vi "Imposta settings grafico.vi"(9 "Reiniz nome plot":bool, 10 "GRAFICO":T1 {"ASSE Y 5"."Decimali" min=0 max=6; "ASSE Y 4"."Decimali" min=0 max=6; "ASSE Y 3"."Decimali" min=0 max=6; "ASSE Y 2"."Decimali" min=0 max=6; "ASSE Y 1"."Decimali" min=0 max=6; "ASSE X 2"."Decimali" min=0 max=6; "ASSE X 1"."Decimali" min=0 max=6}, 11 "XYGraph in":refnum<vi>) -> ()   [LabVIEW 2019]
uses:
  TypeDef/Definizione_Grafico_REPORT.ctl
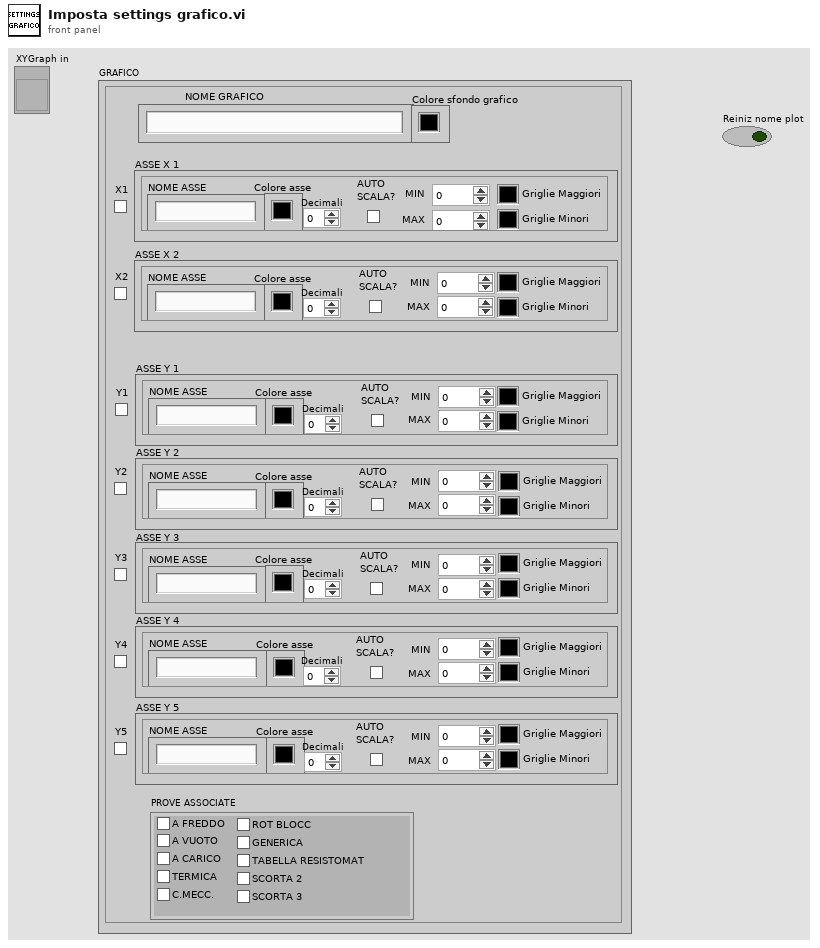
[diagram p1: front panel]
types:
  T1 = typedef "Definizione_Grafico_REPORT.ctl" = cluster{"ASSE X 1":cluster{"NOME ASSE":string, "AUTO\nSCALA?":bool, "MIN":dbl, "MAX":dbl, "Colore asse":u32, "Griglie Maggiori":u32, "Griglie Minori":u32, "Decimali":i8}, "ASSE X 2":cluster{"NOME ASSE":string, "AUTO\nSCALA?":bool, "MIN":dbl, "MAX":dbl, "Colore asse":u32, "Griglie Maggiori":u32, "Griglie Minori":u32, "Decimali":i8}, "ASSE Y 1":cluster{"NOME ASSE":string, "AUTO\nSCALA?":bool, "MIN":dbl, "MAX":dbl, "Colore asse":u32, "Griglie Maggiori":u32, "Griglie Minori":u32, "Decimali":i8}, "ASSE Y 2":cluster{"NOME ASSE":string, "AUTO\nSCALA?":bool, "MIN":dbl, "MAX":dbl, "Colore asse":u32, "Griglie Maggiori":u32, "Griglie Minori":u32, "Decimali":i8}, "ASSE Y 3":cluster{"NOME ASSE":string, "AUTO\nSCALA?":bool, "MIN":dbl, "MAX":dbl, "Colore asse":u32, "Griglie Maggiori":u32, "Griglie Minori":u32, "Decimali":i8}, "ASSE Y 4":cluster{"NOME ASSE":string, "AUTO\nSCALA?":bool, "MIN":dbl, "MAX":dbl, "Colore asse":u32, "Griglie Maggiori":u32, "Griglie Minori":u32, "Decimali":i8}, "X1":bool, "X2":bool, "Y1":bool, "Y2":bool, "Y3":bool, "Y4":bool, "NOME GRAFICO":string, "PROVE ASSOCIATE":cluster{"A FREDDO":bool, "A VUOTO":bool, "A CARICO":bool, "TERMICA":bool, "C.MECC.":bool, "ROT BLOCC":bool, "GENERICA":bool, "TABELLA RESISTOMAT":bool, "SCORTA 2":bool, "SCORTA 3":bool}, "ASSE Y 5":cluster{"NOME ASSE":string, "AUTO\nSCALA?":bool, "MIN":dbl, "MAX":dbl, "Colore asse":u32, "Griglie Maggiori":u32, "Griglie Minori":u32, "Decimali":i8}, "Y5":bool, "Colore sfondo grafico":u32}
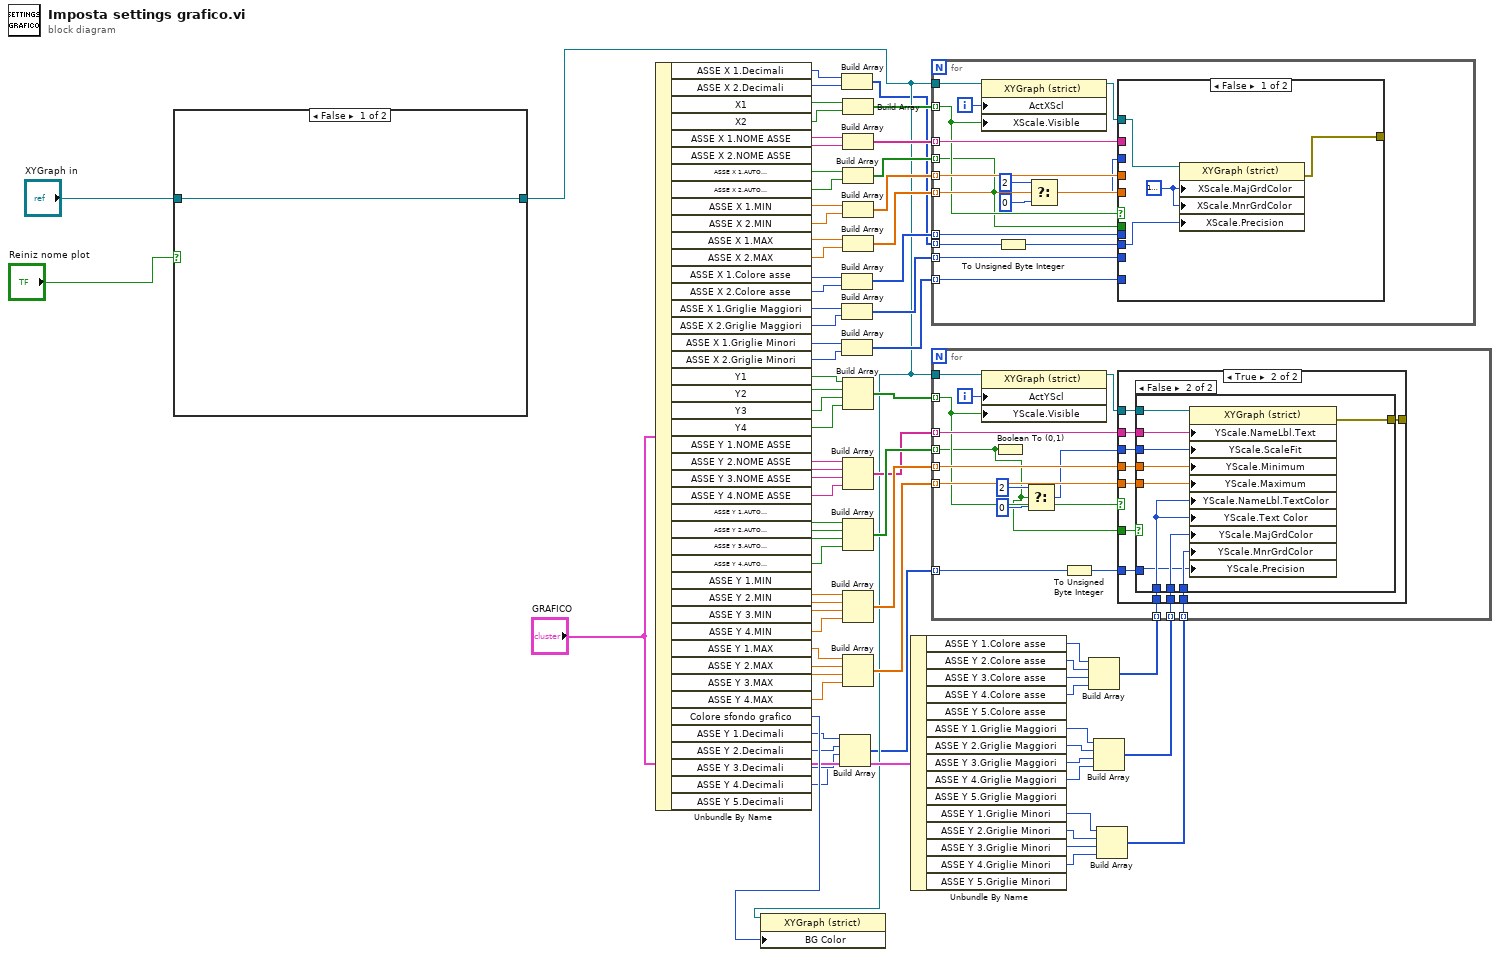
[diagram p0: block diagram]
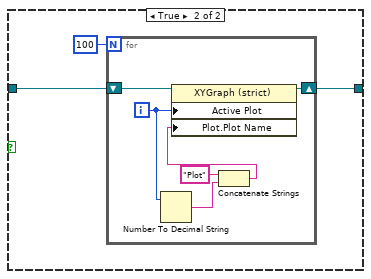
[diagram p2: hidden frame]
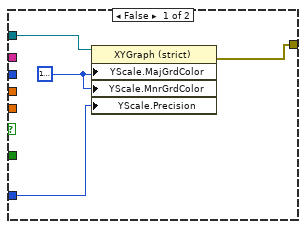
[diagram p3: hidden frame]
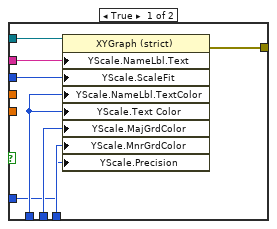
[diagram p4: hidden frame]
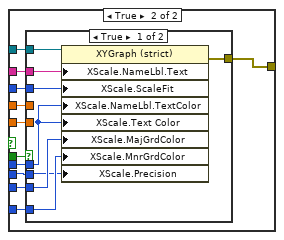
[diagram p5: hidden frame]
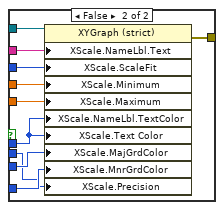
[diagram p6: hidden frame]
diagram:
  n1 = case shown="False" "Reiniz nome plot" {
    tunnel: "XYGraph in" -> [w78 w81]
    tunnel: [w78 w79] -> w7
    frame False {
    }
    frame True {
      n2 = for {
        N: 100 -> [_]
        shift-right: [w82] -> w79
        shift-left: w81 -> [w87]
        i -> [w86]
        n3 = Number To Decimal String(number=w86) -> (decimal integer string=w85:string)  [unwired: 1 in]
        n4 = Concatenate Strings("Plot" ("string"), w85) -> (w83:string)
        n5 = property class="XYGraph (strict)"(reference=w87, "Active Plot"=w86, "Plot.Plot Name"=w83) -> (reference out=w82:refnum<vi>)  [unwired: 1 in, 1 out]
      }
    }
  }
  n6 = Unbundle By Name("GRAFICO") -> ("ASSE X 1.Decimali"=w9:i8, "ASSE X 2.Decimali"=w8:i8, "X1"=w12:bool, "X2"=w13:bool, "ASSE X 1.NOME ASSE"=w15:string, "ASSE X 2.NOME ASSE"=w39:string, "ASSE X 1.AUTO\nSCALA?"=w40:bool, "ASSE X 2.AUTO\nSCALA?"=w41:bool, "ASSE X 1.MIN"=w42:dbl, "ASSE X 2.MIN"=w43:dbl, "ASSE X 1.MAX"=w44:dbl, "ASSE X 2.MAX"=w45:dbl, "ASSE X 1.Colore asse"=w57:u32, "ASSE X 2.Colore asse"=w58:u32, "ASSE X 1.Griglie Maggiori"=w60:u32, "ASSE X 2.Griglie Maggiori"=w61:u32, "ASSE X 1.Griglie Minori"=w63:u32, "ASSE X 2.Griglie Minori"=w64:u32, "Y1"=w59:bool, "Y2"=w20:bool, "Y3"=w21:bool, "Y4"=w22:bool, "ASSE Y 1.NOME ASSE"=w23:string, "ASSE Y 2.NOME ASSE"=w24:string, "ASSE Y 3.NOME ASSE"=w25:string, "ASSE Y 4.NOME ASSE"=w26:string, "ASSE Y 1.AUTO\nSCALA?"=w27:bool, "ASSE Y 2.AUTO\nSCALA?"=w28:bool, "ASSE Y 3.AUTO\nSCALA?"=w29:bool, "ASSE Y 4.AUTO\nSCALA?"=w30:bool, "ASSE Y 1.MIN"=w31:dbl, "ASSE Y 2.MIN"=w32:dbl, "ASSE Y 3.MIN"=w33:dbl, "ASSE Y 4.MIN"=w34:dbl, "ASSE Y 1.MAX"=w35:dbl, "ASSE Y 2.MAX"=w36:dbl, "ASSE Y 3.MAX"=w37:dbl, "ASSE Y 4.MAX"=w38:dbl, "Colore sfondo grafico"=w77:u32, "ASSE Y 1.Decimali"=w1:i8, "ASSE Y 2.Decimali"=w5:i8, "ASSE Y 3.Decimali"=w4:i8, "ASSE Y 4.Decimali"=w3:i8)  [unwired: 1 out]
  n7 = property class="XYGraph (strict)"(reference=w7, "BG Color"=w77) -> ()  [unwired: 1 in, 2 out]
  n8 = Build Array(w1, w5, w4, w3) -> (w2:i8[])
  n9 = Build Array(w9, w8) -> (w6:i8[])
  n10 = Build Array(w57, w58) -> (w51:u32[])
  n11 = Build Array(w60, w61) -> (w62:u32[])
  n12 = Build Array(w63, w64) -> (w65:u32[])
  n13 = Build Array(w12, w13) -> (w14:bool[])
  n14 = Build Array(w15, w39) -> (w16:string[])
  n15 = Build Array(w40, w41) -> (w17:bool[])
  n16 = Build Array(w42, w43) -> (w18:dbl[])
  n17 = Build Array(w44, w45) -> (w19:dbl[])
  n18 = Build Array(w59, w20, w21, w22) -> (w46:bool[])
  n19 = Build Array(w23, w24, w25, w26) -> (w47:string[])
  n20 = Build Array(w27, w28, w29, w30) -> (w48:bool[])
  n21 = Build Array(w31, w32, w33, w34) -> (w49:dbl[])
  n22 = Build Array(w35, w36, w37, w38) -> (w50:dbl[])
  n23 = Unbundle By Name("GRAFICO") -> ("ASSE Y 1.Colore asse"=w53:u32, "ASSE Y 2.Colore asse"=w54:u32, "ASSE Y 3.Colore asse"=w55:u32, "ASSE Y 4.Colore asse"=w56:u32, "ASSE Y 1.Griglie Maggiori"=w66:u32, "ASSE Y 2.Griglie Maggiori"=w67:u32, "ASSE Y 3.Griglie Maggiori"=w68:u32, "ASSE Y 4.Griglie Maggiori"=w69:u32, "ASSE Y 1.Griglie Minori"=w71:u32, "ASSE Y 2.Griglie Minori"=w72:u32, "ASSE Y 3.Griglie Minori"=w73:u32, "ASSE Y 4.Griglie Minori"=w74:u32)  [unwired: 3 out]
  n24 = for {
    tunnel: w14 -> [w97] mode=indexing
    tunnel: w7 -> [w103]
    tunnel: w16 -> [w100] mode=indexing
    tunnel: w17 -> [w92] mode=indexing
    tunnel: w18 -> [w99] mode=indexing
    tunnel: w19 -> [w98] mode=indexing
    tunnel: w51 -> [w96] mode=indexing
    tunnel: w62 -> [w91] mode=indexing
    tunnel: w65 -> [w90] mode=indexing
    tunnel: w6 -> [w89] mode=indexing
    i -> [w102]
    n25 = property class="XYGraph (strict)"(reference=w103, "ActXScl"=w102, "XScale.Visible"=w97) -> (reference out=w101:refnum<vi>)  [unwired: 1 in, 1 out]
    n26 = To Unsigned Byte Integer(number=w89) -> (unsigned 8bit integer=w88:u8)
    n27 = Select(t=i16 2 ("0, 1"), s=w92, f=i16 0 ("0, 1")) -> (s? t:f=w93:i16)
    n28 = case shown="False" w97 {
      tunnel: w101 -> [w107 w118]
      tunnel: w100 -> [_ w117]
      tunnel: w93 -> [_ w116]
      tunnel: w99 -> [_ w115]
      tunnel: w98 -> [_ w114]
      tunnel: w96 -> [_ w113]
      tunnel: w92 -> [_ w112]
      tunnel: w91 -> [_ w111]
      tunnel: w90 -> [_ w110]
      tunnel: w88 -> [w105 w109]
      tunnel: [w104 w108] -> _
      frame False {
        w106 = u32 16777216
        n29 = property class="XYGraph (strict)"(reference=w107, "XScale.MajGrdColor"=w106, "XScale.MnrGrdColor"=w106, "XScale.Precision"=w105) -> (error out=w104:errorcluster)  [unwired: 1 in, 1 out]
      }
      frame True {
        n30 = case shown="True" w112 {
          tunnel: w118 -> [w126 w136]
          tunnel: w117 -> [w125 w135]
          tunnel: w116 -> [w124 w134]
          tunnel: w115 -> [_ w133]
          tunnel: w114 -> [_ w132]
          tunnel: w113 -> [w123 w131]
          tunnel: w111 -> [w122 w130]
          tunnel: w110 -> [w121 w129]
          tunnel: w109 -> [w120 w128]
          tunnel: [w119 w127] -> w108
          frame True {
            n31 = property class="XYGraph (strict)"(reference=w126, "XScale.NameLbl.Text"=w125, "XScale.ScaleFit"=w124, "XScale.NameLbl.TextColor"=w123, "XScale.Text Color"=w123, "XScale.MajGrdColor"=w122, "XScale.MnrGrdColor"=w121, "XScale.Precision"=w120) -> (error out=w119:errorcluster)  [unwired: 1 in, 1 out]
          }
          frame False {
            n32 = property class="XYGraph (strict)"(reference=w136, "XScale.NameLbl.Text"=w135, "XScale.ScaleFit"=w134, "XScale.Minimum"=w133, "XScale.Maximum"=w132, "XScale.NameLbl.TextColor"=w131, "XScale.Text Color"=w131, "XScale.MajGrdColor"=w130, "XScale.MnrGrdColor"=w129, "XScale.Precision"=w128) -> (error out=w127:errorcluster)  [unwired: 1 in, 1 out]
          }
        }
      }
    }
  }
  n33 = Build Array(w53, w54, w55, w56) -> (w52:u32[])
  n34 = Build Array(w66, w67, w68, w69) -> (w70:u32[])
  n35 = Build Array(w71, w72, w73, w74) -> (w75:u32[])
  n36 = for {
    tunnel: w46 -> [w146] mode=indexing
    tunnel: w7 -> [w152]
    tunnel: w47 -> [w149] mode=indexing
    tunnel: w48 -> [w141] mode=indexing
    tunnel: w49 -> [w148] mode=indexing
    tunnel: w50 -> [w147] mode=indexing
    tunnel: w52 -> [w145] mode=indexing
    tunnel: w70 -> [w140] mode=indexing
    tunnel: w75 -> [w139] mode=indexing
    tunnel: w2 -> [w137] mode=indexing
    i -> [w151]
    n37 = property class="XYGraph (strict)"(reference=w152, "ActYScl"=w151, "YScale.Visible"=w146) -> (reference out=w150:refnum<vi>)  [unwired: 1 in, 1 out]
    n38 = Boolean To (0,1)(Boolean=w141) -> ()  [unwired: 1 out]
    n39 = Select(t=i16 2 ("0, 1"), s=w141, f=i16 0 ("0, 1")) -> (s? t:f=w142:i16)
    n40 = To Unsigned Byte Integer(number=w137) -> (unsigned 8bit integer=w138:u8)
    n41 = case shown="True" w146 {
      tunnel: w150 -> [w156 w167]
      tunnel: w149 -> [_ w166]
      tunnel: w142 -> [_ w165]
      tunnel: w148 -> [_ w164]
      tunnel: w147 -> [_ w163]
      tunnel: w145 -> [_ w162]
      tunnel: w141 -> [_ w161]
      tunnel: w140 -> [_ w160]
      tunnel: w139 -> [_ w159]
      tunnel: w138 -> [w154 w158]
      tunnel: [w153 w157] -> _
      frame False {
        w155 = u32 16777216
        n42 = property class="XYGraph (strict)"(reference=w156, "YScale.MajGrdColor"=w155, "YScale.MnrGrdColor"=w155, "YScale.Precision"=w154) -> (error out=w153:errorcluster)  [unwired: 1 in, 1 out]
      }
      frame True {
        n43 = case shown="False" w161 {
          tunnel: w167 -> [w175 w185]
          tunnel: w166 -> [w174 w184]
          tunnel: w165 -> [w173 w183]
          tunnel: w164 -> [_ w182]
          tunnel: w163 -> [_ w181]
          tunnel: w162 -> [w172 w180]
          tunnel: w160 -> [w171 w179]
          tunnel: w159 -> [w170 w178]
          tunnel: w158 -> [w169 w177]
          tunnel: [w168 w176] -> w157
          frame True {
            n44 = property class="XYGraph (strict)"(reference=w175, "YScale.NameLbl.Text"=w174, "YScale.ScaleFit"=w173, "YScale.NameLbl.TextColor"=w172, "YScale.Text Color"=w172, "YScale.MajGrdColor"=w171, "YScale.MnrGrdColor"=w170, "YScale.Precision"=w169) -> (error out=w168:errorcluster)  [unwired: 1 in, 1 out]
          }
          frame False {
            n45 = property class="XYGraph (strict)"(reference=w185, "YScale.NameLbl.Text"=w184, "YScale.ScaleFit"=w183, "YScale.Minimum"=w182, "YScale.Maximum"=w181, "YScale.NameLbl.TextColor"=w180, "YScale.Text Color"=w180, "YScale.MajGrdColor"=w179, "YScale.MnrGrdColor"=w178, "YScale.Precision"=w177) -> (error out=w176:errorcluster)  [unwired: 1 in, 1 out]
          }
        }
      }
    }
  }
